vi "Untitled 1.vi"() -> ()   [LabVIEW 2017]
panel:
  out "x+y":dbl
  in  "x":dbl
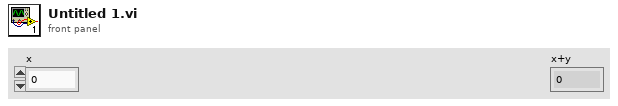
[diagram p1: front panel]
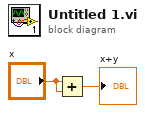
[diagram p0: block diagram]
diagram:
  n1 = Add(x="x", y="x") -> (x+y=→"x+y":dbl)
